vi "Reset Counter.vi"(3 "Reset":bool) -> (1 "Counter":i32)   [LabVIEW 2016, in "Control Experiment.lvclass"]
uses:
  Control Experiment.lvclass
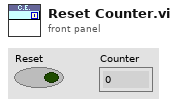
[diagram p1: front panel]
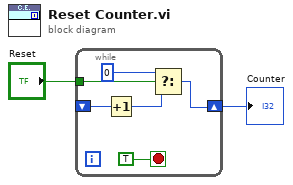
[diagram p0: block diagram]
diagram:
  n1 = while {
    shift-right: [w5] -> w2
    shift-left: _ -> [w6]
    tunnel: "Reset" -> [w8]
    stop <- TRUE stop-if-true
    n2 = Increment(x=w6) -> (x+1=w3:i32)
    n3 = Select(t=0 ("Append Index"), s=w8, f=w3) -> (s? t:f=w5:i32)
  }
  "Counter" <- w2
